vi "LoadApplicationConfig.vi"(8 "error in (no error)":errorcluster) -> (0 "error out":errorcluster, 2 "Config Cluster":T1, 3 "refnum out":T2)   [LabVIEW 2026]
uses:
  <vilib>/Utility/config.llb/Config Data RefNum.ctl
  controls/Vibration_Monitor_Config.ctl
  <vilib>/Utility/config.llb/Read Key (String).vi
  <vilib>/Utility/config.llb/NI_LVConfig.lvlib
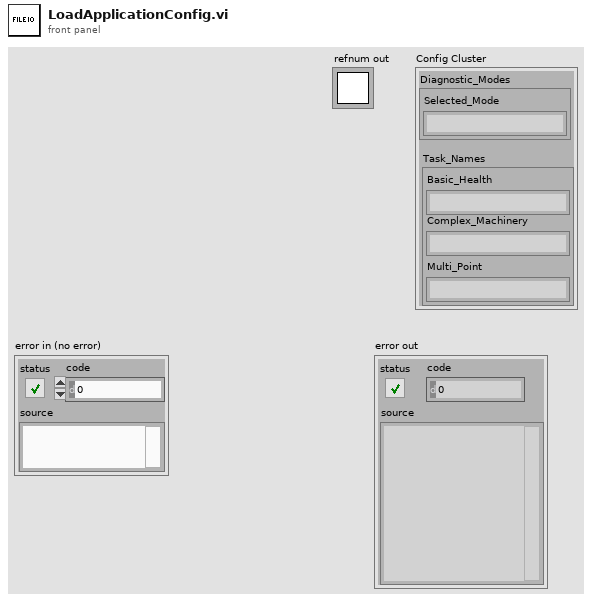
[diagram p1: front panel]
types:
  T1 = typedef "Vibration_Monitor_Config.ctl" = cluster{"Diagnostic_Modes":cluster{"Selected_Mode":string}, "Task_Names":cluster{"Basic_Health":string, "Complex_Machinery":string, "Multi_Point":string}}
  T2 = typedef "NI_LVConfig.lvlib/Config Data RefNum.ctl" = refnum<k1>
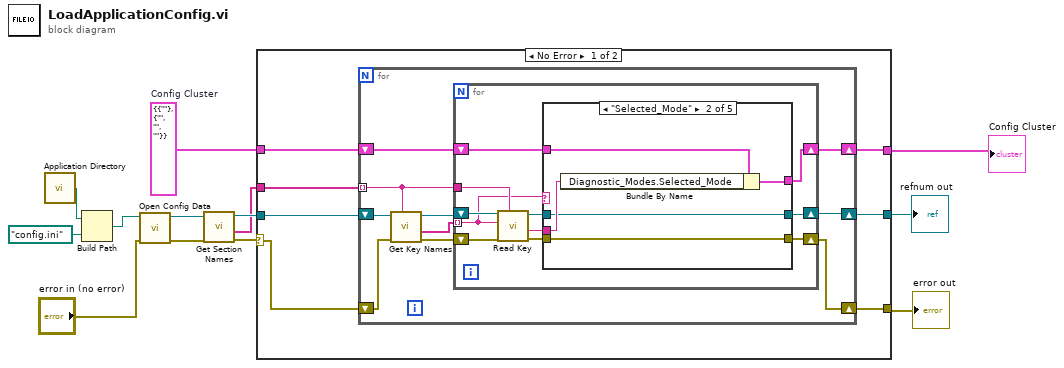
[diagram p0: block diagram]
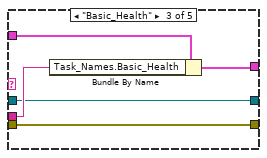
[diagram p3: hidden frame]
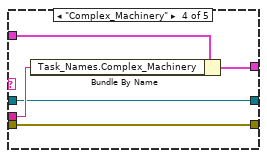
[diagram p4: hidden frame]
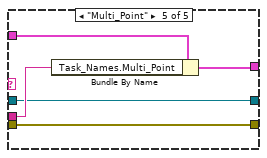
[diagram p5: hidden frame]
diagram:
  w2 = T1 {"Diagnostic_Modes"={"Selected_Mode"=""}, "Task_Names"={"Basic_Health"="", "Complex_Machinery"="", "Multi_Point"=""}}  # Config Cluster
  n1 = call <vilib>:"Application Directory.vi"() -> ("Application Directory"=w12:path)
  n2 = Build Path(base path=w12, name or relative path=path "config.ini") -> (appended path=w13:path)
  n3 = call <vilib>:"Open Config Data.vi"("error in (no error)"="error in (no error)", "configuration file path"=w13) -> ("error out"=w9:errorcluster, "refnum"=w10:T2)  [unwired: 7 in, 1 out]
  n4 = call <vilib>:"Get Section Names.vi"("error in (no error)"=w9, "refnum"=w10) -> ("error out"=w6:errorcluster, "section names"=w4:string[], "refnum out"=w5:T2)  [unwired: 7 in]
  n5 = case shown="No Error" w6 {
    selector: w6 -> [w19 w67]
    tunnel: [w17 w67] -> w8
    tunnel: w5 -> [w20 w66]
    tunnel: w4 -> [w18 _]
    tunnel: [w16 w66] -> w3
    tunnel: w2 -> [w15 w65]
    tunnel: [w14 w65] -> w1
    frame No Error {
      n6 = for {
        tunnel: w18 -> [w22] mode=indexing
        shift-right: [w26] -> w17
        shift-left: w19 -> [w29]
        shift-right: [w24] -> w16
        shift-left: w20 -> [w30]
        shift-right: [w21] -> w14
        shift-left: w15 -> [w23]
        n7 = call <vilib>:"Get Key Names.vi"("section"=w22, "error in (no error)"=w29, "refnum"=w30) -> ("error out"=w28:errorcluster, "key names"=w25:string[], "refnum out"=w27:T2)  [unwired: 5 in, 1 out]
        n8 = for {
          shift-right: [w33] -> w26
          shift-left: w28 -> [w35]
          tunnel: w25 -> [w39] mode=indexing
          shift-right: [w31] -> w24
          shift-left: w27 -> [w41]
          tunnel: w22 -> [w40]
          shift-right: [w37] -> w21
          shift-left: w23 -> [w36]
          n9 = call-poly <vilib>:"Read Key.vi"("section"=w40, "error in (no error)"=w35, "key"=w39, "refnum"=w41) -> ("error out"=w34:errorcluster, "value"=w38:string, "refnum out"=w32:T2)  [unwired: 4 in, 1 out]
          n10 = case shown="\"Selected_Mode\"" w39 {
            tunnel: w38 -> [_ w49 w54 w59 w64]
            tunnel: [w44 w48 w53 w58 w63] -> w37
            tunnel: w36 -> [w44 w47 w52 w57 w62]
            tunnel: w34 -> [w43 w46 w51 w56 w61]
            tunnel: [w43 w46 w51 w56 w61] -> w33
            tunnel: w32 -> [w42 w45 w50 w55 w60]
            tunnel: [w42 w45 w50 w55 w60] -> w31
            frame Default {
            }
            frame "Selected_Mode" {
              n11 = Bundle By Name(cluster=w47, "Diagnostic_Modes.Selected_Mode"=w49) -> (w48:T1)
            }
            frame "Basic_Health" {
              n12 = Bundle By Name(cluster=w52, "Task_Names.Basic_Health"=w54) -> (w53:T1)
            }
            frame "Complex_Machinery" {
              n13 = Bundle By Name(cluster=w57, "Task_Names.Complex_Machinery"=w59) -> (w58:T1)
            }
            frame "Multi_Point" {
              n14 = Bundle By Name(cluster=w62, "Task_Names.Multi_Point"=w64) -> (w63:T1)
            }
          }
        }
      }
    }
    frame Error {
    }
  }
  "error out" <- w8
  "refnum out" <- w3
  "Config Cluster" <- w1
